vi "lv_mysql_conn_init_client_data.vi"(8 "error in (no error)":errorcluster, 10 "Authentication":T1, 11 "Server Init Data":T2 {"Server Status" format="%.0x"; "Server Languague" format="%.0x"; "Server Capabilities" format="%.0x"}) -> (0 "error out":errorcluster, 3 "TCPIP Data":u8[](array[numeric]))   [LabVIEW 2020]
uses:
  Control/server_init_data.ctl
  Control/mysql_authentication.ctl
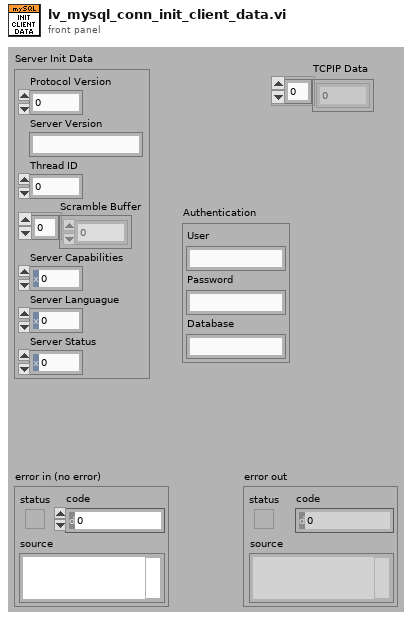
[diagram p1: front panel]
types:
  T1 = typedef "mysql_authentication.ctl" = cluster{"User":string, "Password":string, "Database":string}
  T2 = typedef "server_init_data.ctl" = cluster{"Protocol Version":u8, "Server Version":string, "Thread ID":u32, "Scramble Buffer":u8[], "Server Capabilities":u16, "Server Languague":u8, "Server Status":u16}
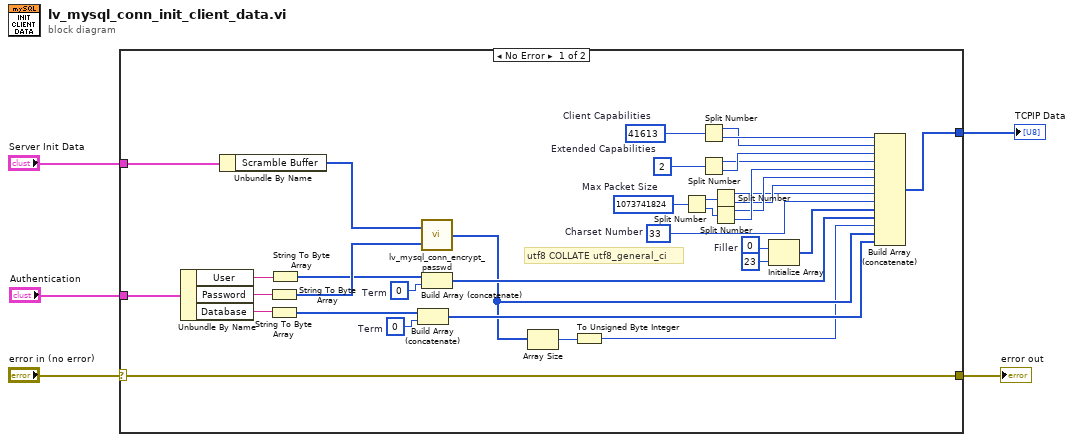
[diagram p0: block diagram]
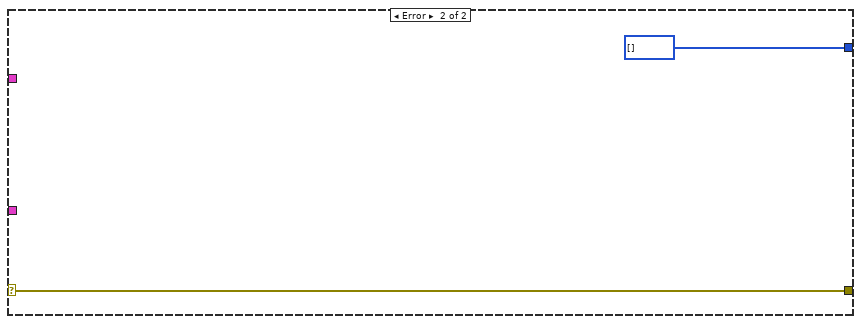
[diagram p2: hidden frame]
diagram:
  n1 = case shown="No Error" "error in (no error)" {
    selector: "error in (no error)" -> [w40 w42]
    tunnel: [w40 w42] -> w5
    tunnel: "Server Init Data" -> [w39 _]
    tunnel: [w21 u8[] [] ("TCPIP Data 2")] -> w2
    tunnel: "Authentication" -> [w24 _]
    frame No Error {
      w11 = u8 0  # Term
      w12 = u8 0  # Term
      w16 = u8 0  # Filler
      w34 = u16 2  # Extended Capabilities
      w38 = u16 41613  # Client Capabilities
      w25 = u8 33  # Charset Number
      w35 = u32 1073741824  # Max Packet Size
      # "utf8 COLLATE utf8_general_ci"
      n2 = Unbundle By Name(w24) -> ("User"=w23:string, "Password"=w20:string, "Database"=w22:string)
      n3 = Unbundle By Name(w39) -> ("Scramble Buffer"=w19:u8[])
      n4 = String To Byte Array(string=w20) -> (unsigned byte array=w18:u8[])
      n5 = String To Byte Array(string=w22) -> (unsigned byte array=w10:u8[])
      n6 = String To Byte Array(string=w23) -> (unsigned byte array=w14:u8[])
      n7 = Build Array (concatenate)(w10, w11) -> (w9:u8[])
      n8 = call "lv_mysql_conn_encrypt_passwd.vi"("Data"=w18, "Scramble"=w19) -> ("SHA1 Data"=w8:u8[])
      n9 = Build Array (concatenate)(w14, w12) -> (w13:u8[])
      n10 = Array Size(array=w8) -> (size(s)=w7:i32)
      n11 = To Unsigned Byte Integer(number=w7) -> (unsigned 8bit integer=w6:u8)
      n12 = Split Number(x=w35) -> (hi(x)=w36:u16, lo(x)=w37:u16)
      n13 = Split Number(x=w38) -> (hi(x)=w32:u8, lo(x)=w33:u8)
      n14 = Split Number(x=w34) -> (hi(x)=w30:u8, lo(x)=w31:u8)
      n15 = Split Number(x=w36) -> (hi(x)=w26:u8, lo(x)=w27:u8)
      n16 = Split Number(x=w37) -> (hi(x)=w28:u8, lo(x)=w29:u8)
      n17 = Initialize Array(w16, 23 ("dimension size")) -> (w15:u8[])
      n18 = Build Array (concatenate)(w33, w32, w31, w30, w29, w28, w27, w26, w25, w15, w13, w6, w8, w9) -> (w21:u8[])
    }
    frame Error {
    }
  }
  "error out" <- w5
  "TCPIP Data" <- w2
